vi "Control panel loop.vi"   [LabVIEW 2016]
doc: "This VI is used to convert the flags into events."
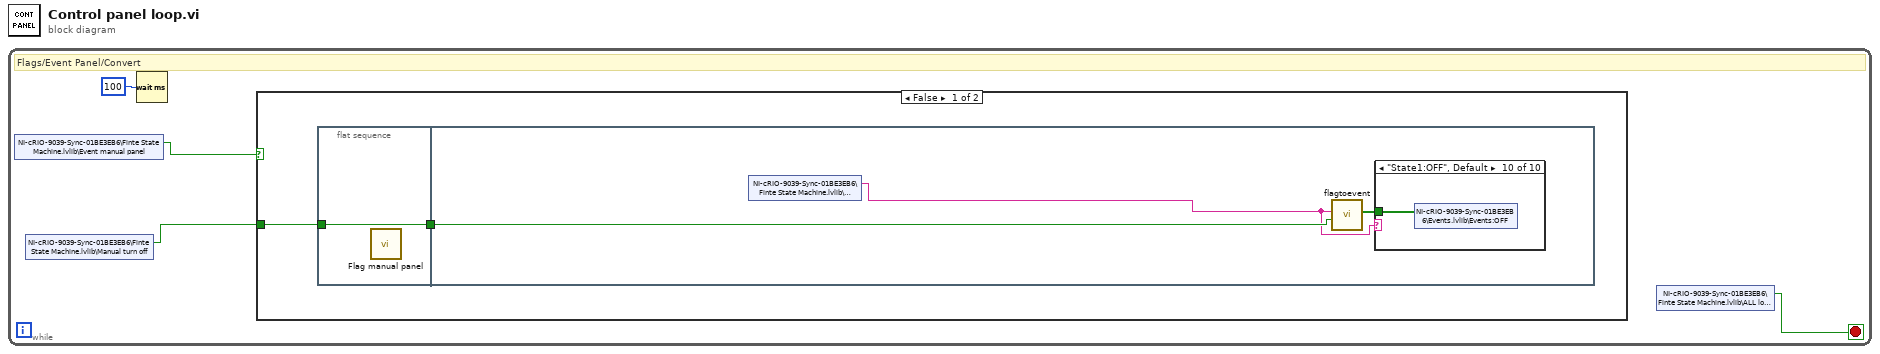
[diagram p0: block diagram]
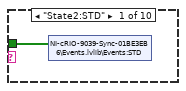
[diagram p2: hidden frame]
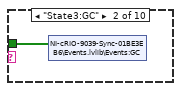
[diagram p3: hidden frame]
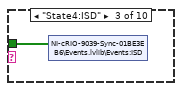
[diagram p4: hidden frame]
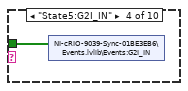
[diagram p5: hidden frame]
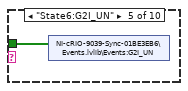
[diagram p6: hidden frame]
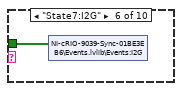
[diagram p7: hidden frame]
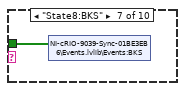
[diagram p8: hidden frame]
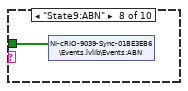
[diagram p9: hidden frame]
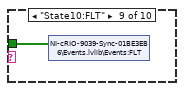
[diagram p10: hidden frame]
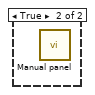
[diagram p11: hidden frame]
diagram:
  n1 = while {
    stop <- w3 stop-if-true
    # "Flags/Event Panel/Convert"
    n2 = shared-variable "NI-cRIO-9039-Sync-01BE3EB6\\Finte State Machine.lvlib\\Event manual panel"() -> (w2:bool)  [unwired: 1 in, 1 out]
    n3 = shared-variable "NI-cRIO-9039-Sync-01BE3EB6\\Finte State Machine.lvlib\\Manual turn off"() -> (w1:bool)  [unwired: 1 in, 1 out]
    n4 = Wait (ms)(milliseconds to wait=u32 100) -> ()  [unwired: 1 out]
    n5 = case shown="False" w2 {
      tunnel: w1 -> [w6 _]
      frame False {
        n6 = flat-sequence {
          tunnel: w6 -> [w7]
          tunnel: [w7] -> w5
          tunnel: w5 -> [w10]
          frame #0 {
            n7 = call "Flag manual panel.vi"() -> ()  [unwired: 12 in]
          }
          frame #1 {
            n8 = shared-variable "NI-cRIO-9039-Sync-01BE3EB6\\Finte State Machine.lvlib\\Current state"() -> (w8:string)  [unwired: 1 in, 1 out]
            n9 = call "flagtoevent.vi"("M_OFF"=w10, "Pre_state"=w8) -> ("Event"=w9:bool[])  [unwired: 9 in]
            n10 = case shown="\"State1:OFF\", Default" w8 {
              tunnel: w9 -> [w11 w12 w13 w14 w15 w16 w17 w18 w19 w20]
              frame "State2:STD" {
                n11 = shared-variable "NI-cRIO-9039-Sync-01BE3EB6\\Events.lvlib\\Events:STD"(w11) -> ()  [unwired: 1 in, 1 out]
              }
              frame "State3:GC" {
                n12 = shared-variable "NI-cRIO-9039-Sync-01BE3EB6\\Events.lvlib\\Events:GC"(w12) -> ()  [unwired: 1 in, 1 out]
              }
              frame "State4:ISD" {
                n13 = shared-variable "NI-cRIO-9039-Sync-01BE3EB6\\Events.lvlib\\Events:ISD"(w13) -> ()  [unwired: 1 in, 1 out]
              }
              frame "State5:G2I_IN" {
                n14 = shared-variable "NI-cRIO-9039-Sync-01BE3EB6\\Events.lvlib\\Events:G2I_IN"(w14) -> ()  [unwired: 1 in, 1 out]
              }
              frame "State6:G2I_UN" {
                n15 = shared-variable "NI-cRIO-9039-Sync-01BE3EB6\\Events.lvlib\\Events:G2I_UN"(w15) -> ()  [unwired: 1 in, 1 out]
              }
              frame "State7:I2G" {
                n16 = shared-variable "NI-cRIO-9039-Sync-01BE3EB6\\Events.lvlib\\Events:I2G"(w16) -> ()  [unwired: 1 in, 1 out]
              }
              frame "State8:BKS" {
                n17 = shared-variable "NI-cRIO-9039-Sync-01BE3EB6\\Events.lvlib\\Events:BKS"(w17) -> ()  [unwired: 1 in, 1 out]
              }
              frame "State9:ABN" {
                n18 = shared-variable "NI-cRIO-9039-Sync-01BE3EB6\\Events.lvlib\\Events:ABN"(w18) -> ()  [unwired: 1 in, 1 out]
              }
              frame "State10:FLT" {
                n19 = shared-variable "NI-cRIO-9039-Sync-01BE3EB6\\Events.lvlib\\Events:FLT"(w19) -> ()  [unwired: 1 in, 1 out]
              }
              frame "State1:OFF", Default {
                n20 = shared-variable "NI-cRIO-9039-Sync-01BE3EB6\\Events.lvlib\\Events:OFF"(w20) -> ()  [unwired: 1 in, 1 out]
              }
            }
          }
        }
      }
      frame True {
        n21 = call "Manual panel.vi"() -> ()  [unwired: 12 in]
      }
    }
    n22 = shared-variable "NI-cRIO-9039-Sync-01BE3EB6\\Finte State Machine.lvlib\\ALL loop stop"() -> (w3:bool)  [unwired: 1 in, 1 out]
  }
